vi "SV Refnum.vi"(11 "variable reference in":refnum<k21>) -> (3 "shared variable refnum out":refnum<k21>)   [LabVIEW 2018, in "Dynamic Shared Variables.lvlib"]
uses:
  Dynamic Shared Variables.lvlib
panel:
  out "match + rest of string":string
  out "string":string="\\\\.\\sv_alarm_example\\my_number"
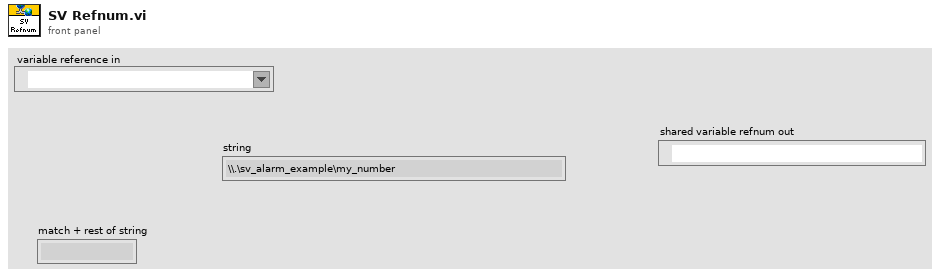
[diagram p1: front panel]
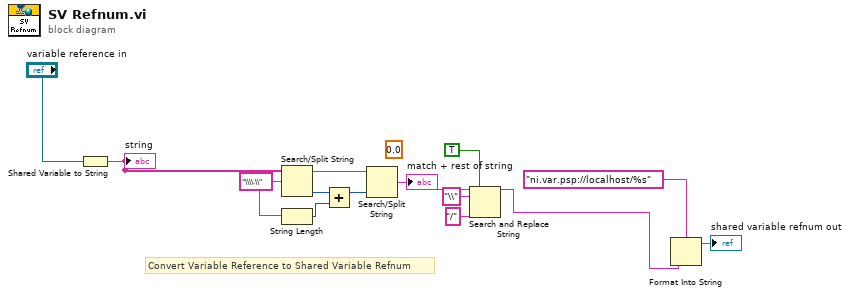
[diagram p0: block diagram]
diagram:
  w11 = "\\\\.\\" ("search string/char (-)")
  (unwired) 0.0
  # "Convert Variable Reference to Shared Variable Refnum"
  n1 = Shared Variable to String(1:"variable reference in") -> (0:w12:string)
  "string" <- w12
  n2 = Search/Split String(string=w12, search string/char (-)=w11) -> (offset of match=w10:i32)  [unwired: 1 in, 2 out]
  n3 = String Length(string=w11) -> (length=w8:i32)
  n4 = Add(x=w10, y=w8) -> (x+y=w9:i32)
  n5 = Search/Split String(string=w12, offset (0)=w9) -> (match + rest of string=w7:string)  [unwired: 1 in, 2 out]
  "match + rest of string" <- w7
  n6 = Search and Replace String(replace all?=TRUE ("replace all? (F)"), input string=w7, search string="\\", replace string="/" ("replace string (\"\")")) -> (result string=w3:string)  [unwired: 4 in, 3 out]
  n7 = Format Into String(format string="ni.var.psp://localhost/%s", w3) -> (resulting string=→"shared variable refnum out":string)  [unwired: 2 in, 1 out]
